vi "getApplicationPath.vi"(8 "error in (no error)":errorcluster) -> (0 "error out":errorcluster, 2 "ApplicationPath":path)   [LabVIEW 2011]
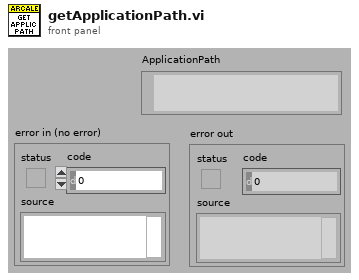
[diagram p1: front panel]
types:
  T1 = enum32{"invalid app kind", "Development System", "Run Time System", "Student Edition", "Embedded LabVIEW", "Evaluation", "Custom"}
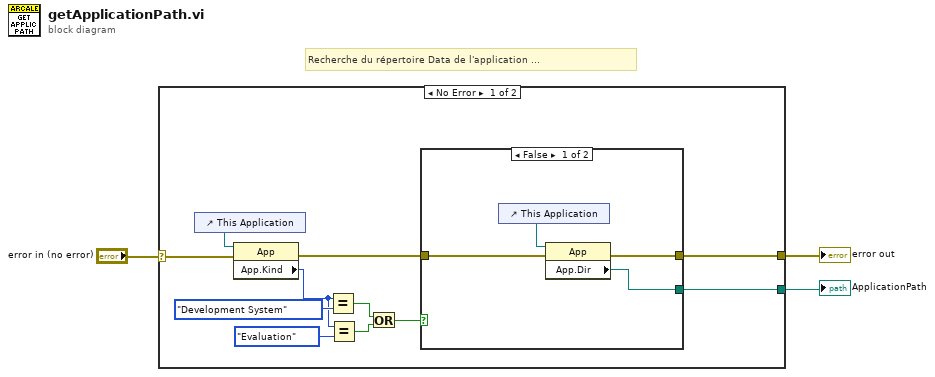
[diagram p0: block diagram]
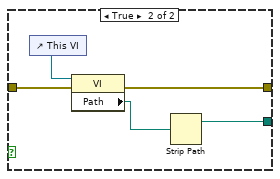
[diagram p2: hidden frame]
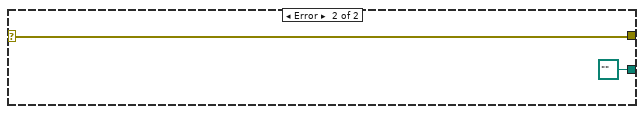
[diagram p3: hidden frame]
diagram:
  # "Recherche du répertoire Data de l'application ..."
  n1 = case shown="No Error" "error in (no error)" {
    selector: "error in (no error)" -> [w11 w24]
    tunnel: [w9 path "" ("appended path")] -> w3
    tunnel: [w10 w24] -> w1
    frame No Error {
      n2 = control-ref of="This Application"() -> (w14:refnum<vi>)
      n3 = property class="App"(reference=w14, error in=w11) -> (error out=w12:errorcluster, "App.Kind"=w8:T1)  [unwired: 1 out]
      n4 = Equal?(x=w8, y=T1."Development System") -> (x = y?=w5:bool)
      n5 = Equal?(x=w8, y=T1."Evaluation") -> (x = y?=w6:bool)
      n6 = Or(x=w5, y=w6) -> (x .or. y?=w4:bool)
      n7 = case shown="False" w4 {
        tunnel: [w17 w21] -> w9
        tunnel: w12 -> [w16 w20]
        tunnel: [w15 w19] -> w10
        frame False {
          n8 = control-ref of="This Application"() -> (w18:refnum<vi>)
          n9 = property class="App"(reference=w18, error in=w16) -> (error out=w15:errorcluster, "App.Dir"=w17:path)  [unwired: 1 out]
        }
        frame True {
          n10 = control-ref of="This VI"() -> (w22:refnum<vi>)
          n11 = property class="VI"(reference=w22, error in=w20) -> (error out=w19:errorcluster, "Path"=w23:path)  [unwired: 1 out]
          n12 = Strip Path(path=w23) -> (stripped path=w21:path)  [unwired: 1 out]
        }
      }
    }
    frame Error {
    }
  }
  "error out" <- w1
  "ApplicationPath" <- w3
